vi "File_StingToPath.vi"(11 "Description":string) -> (3 "Path":path)   [LabVIEW 2012]
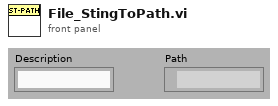
[diagram p1: front panel]
types:
  T1 = enum32{"invalid OS target", "Mac OS", "Windows 3.1", "Windows 95/NT", "Solaris 1", "Solaris 2", "HP-UX", "PowerMAX", "Linux", "Irix", "Rhapsody", "BeOS", "AIX", "OSF1", "VxWorks", "PharLap", "Carbon", "RTX", "Windows x64", "Linux x64"}
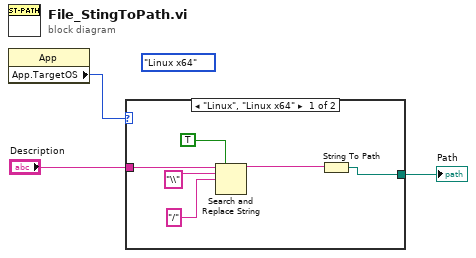
[diagram p0: block diagram]
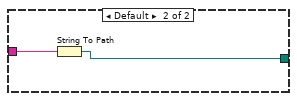
[diagram p2: hidden frame]
diagram:
  (unwired) T1."Linux x64" ("Application:Target:Operating System")
  n1 = property class="App"() -> ("App.TargetOS"=w1:T1)  [unwired: 2 in, 2 out]
  n2 = case shown="\"Linux\", \"Linux x64\"" w1 {
    tunnel: [w9 w11] -> w3
    tunnel: "Description" -> [w8 w10]
    frame "Linux", "Linux x64" {
      n3 = Search and Replace String(replace all?=TRUE ("replace all? (F)"), input string=w8, search string="\\", replace string="/" ("replace string (\"\")")) -> (result string=w7:string)  [unwired: 4 in, 3 out]
      n4 = String To Path(string=w7) -> (path=w9:path)
    }
    frame Default {
      n5 = String To Path(string=w10) -> (path=w11:path)
    }
  }
  "Path" <- w3
